vi "Terminal-Alert-DriverSystem.vi"(11 "动力子系统设备信息":T1) -> (3 "动力子系统设备信息输出":T1)   [LabVIEW 2014]
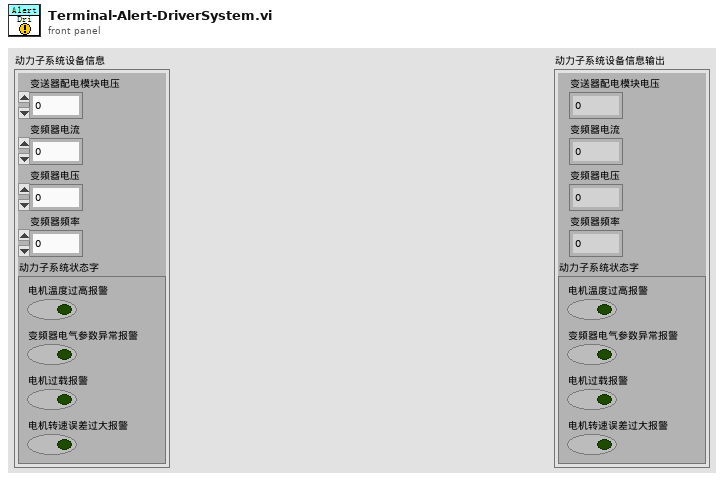
[diagram p1: front panel]
types:
  T1 = cluster{"变送器配电模块电压":u16, "变频器电流":u16, "变频器电压":u16, "变频器频率":u16, "动力子系统状态字":cluster{"电机温度过高报警":bool, "变频器电气参数异常报警":bool, "电机过载报警":bool, "电机转速误差过大报警":bool}}
  T2 = cluster{"报警级别":string, "报警系统":string, "报警详情":string, "备注":string}
  T3 = cluster{"电机温度过高报警":bool, "变频器电气参数异常报警":bool, "电机过载报警":bool, "电机转速误差过大报警":bool}
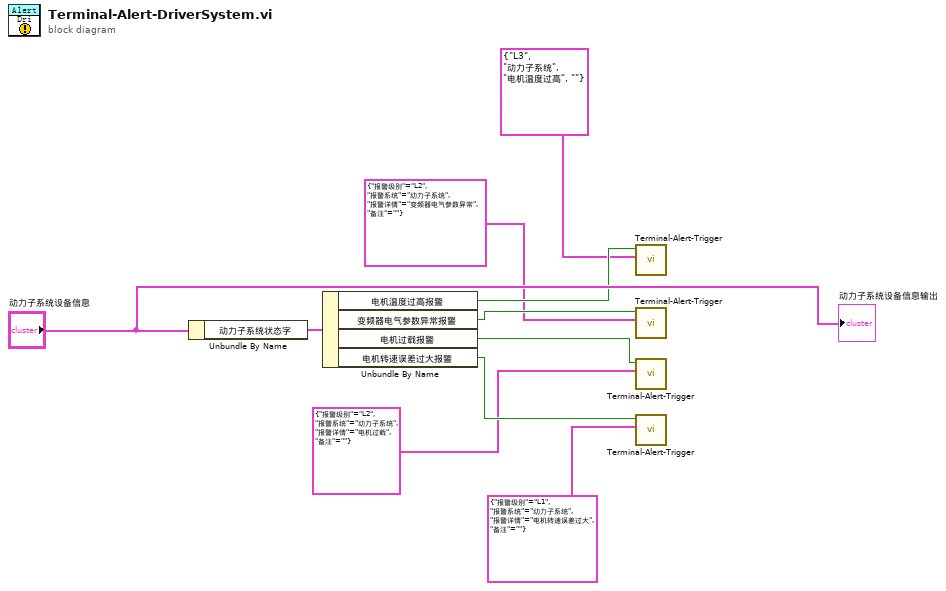
[diagram p0: block diagram]
diagram:
  n1 = Unbundle By Name("动力子系统设备信息") -> ("动力子系统状态字"=w9:T3)
  n2 = Unbundle By Name(w9) -> ("电机温度过高报警"=w8:bool, "变频器电气参数异常报警"=w6:bool, "电机过载报警"=w5:bool, "电机转速误差过大报警"=w4:bool)
  n3 = call "Terminal-Alert-Trigger.vi"("报警信息"=T2 {"报警级别"="L3", "报警系统"="动力子系统", "报警详情"="电机温度过高", "备注"=""}, "是否触发(T)"=w8) -> ()  [unwired: 9 in, 1 out]
  n4 = call "Terminal-Alert-Trigger.vi"("报警信息"=T2 {"报警级别"="L2", "报警系统"="动力子系统", "报警详情"="变频器电气参数异常", "备注"=""}, "是否触发(T)"=w6) -> ()  [unwired: 9 in, 1 out]
  n5 = call "Terminal-Alert-Trigger.vi"("报警信息"=T2 {"报警级别"="L2", "报警系统"="动力子系统", "报警详情"="电机过载", "备注"=""}, "是否触发(T)"=w5) -> ()  [unwired: 9 in, 1 out]
  n6 = call "Terminal-Alert-Trigger.vi"("报警信息"=T2 {"报警级别"="L1", "报警系统"="动力子系统", "报警详情"="电机转速误差过大", "备注"=""}, "是否触发(T)"=w4) -> ()  [unwired: 9 in, 1 out]
  "动力子系统设备信息输出" <- "动力子系统设备信息"
